vi "Dialouge Box Continue.vi"() -> ()   [LabVIEW 2024]
panel:
  out "String 2":string
  in  "String":string
  in  "y":u32
  out "Boolean":bool
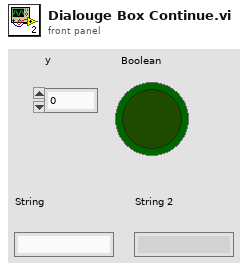
[diagram p1: front panel]
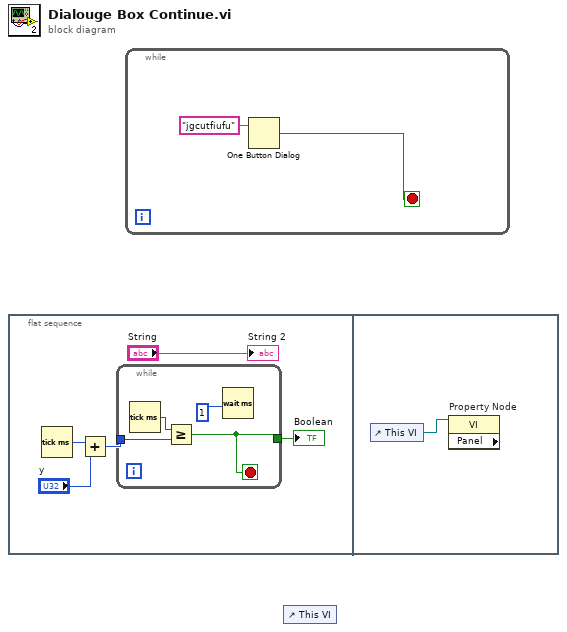
[diagram p0: block diagram]
diagram:
  n1 = flat-sequence {
    frame #0 {
      n2 = Tick Count (ms)() -> (millisecond timer value=w5:u32)
      n3 = Add(x=w5, y="y") -> (x+y=w4:u32)
      n4 = while {
        tunnel: w4 -> [w8]
        tunnel: [w6] -> w3
        stop <- w6 stop-if-true
        n5 = Tick Count (ms)() -> (millisecond timer value=w9:u32)
        n6 = Greater Or Equal?(x=w9, y=w8) -> (x >= y?=w6:bool)
        n7 = Wait (ms)(milliseconds to wait=u32 1) -> ()  [unwired: 1 out]
      }
      "Boolean" <- w3
      "String 2" <- "String"
    }
    frame #1 {
      n8 = control-ref of="This VI"() -> (w10:refnum<vi>)
      n9 = property on="Property Node" class="VI" props=["Panel"](reference=w10) -> ()  [unwired: 1 in, 3 out]
    }
  }
  n10 = while {
    stop <- w12 stop-if-true
    n11 = One Button Dialog(message="jgcutfiufu") -> (true=w12:bool)  [unwired: 1 in]
  }
  n12 = control-ref of="This VI"() -> ()  [unwired: 1 out]
